vi "GOOP_RecompileDialog.vi"(5 "error in (no error)":errorcluster) -> (19 "error out":errorcluster)   [LabVIEW 2020]
panel:
  out "Progress":u8(slide) scale=0.0..100.0
  in  "_Cancel":bool
  in  "_Recompile":bool
  # "Open GOOP\nDevelopment Suite"
  # "OpenGDS needs to be re-compiled. If you re-compile the OpenGDS it will load faster and be more stable. Do you want to re-compile now?\nIt will take some time to re-compile OpenGDS."
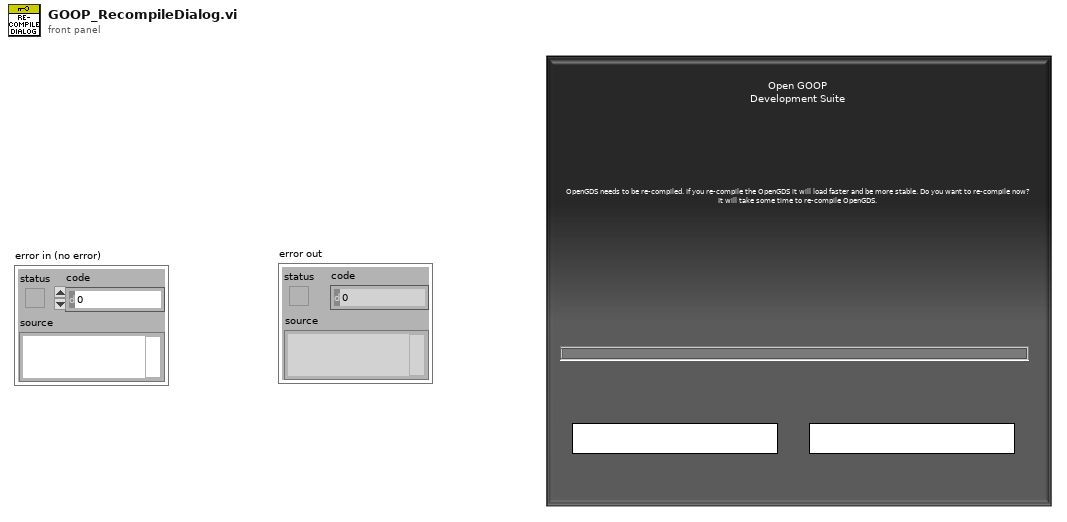
[diagram p1: front panel]
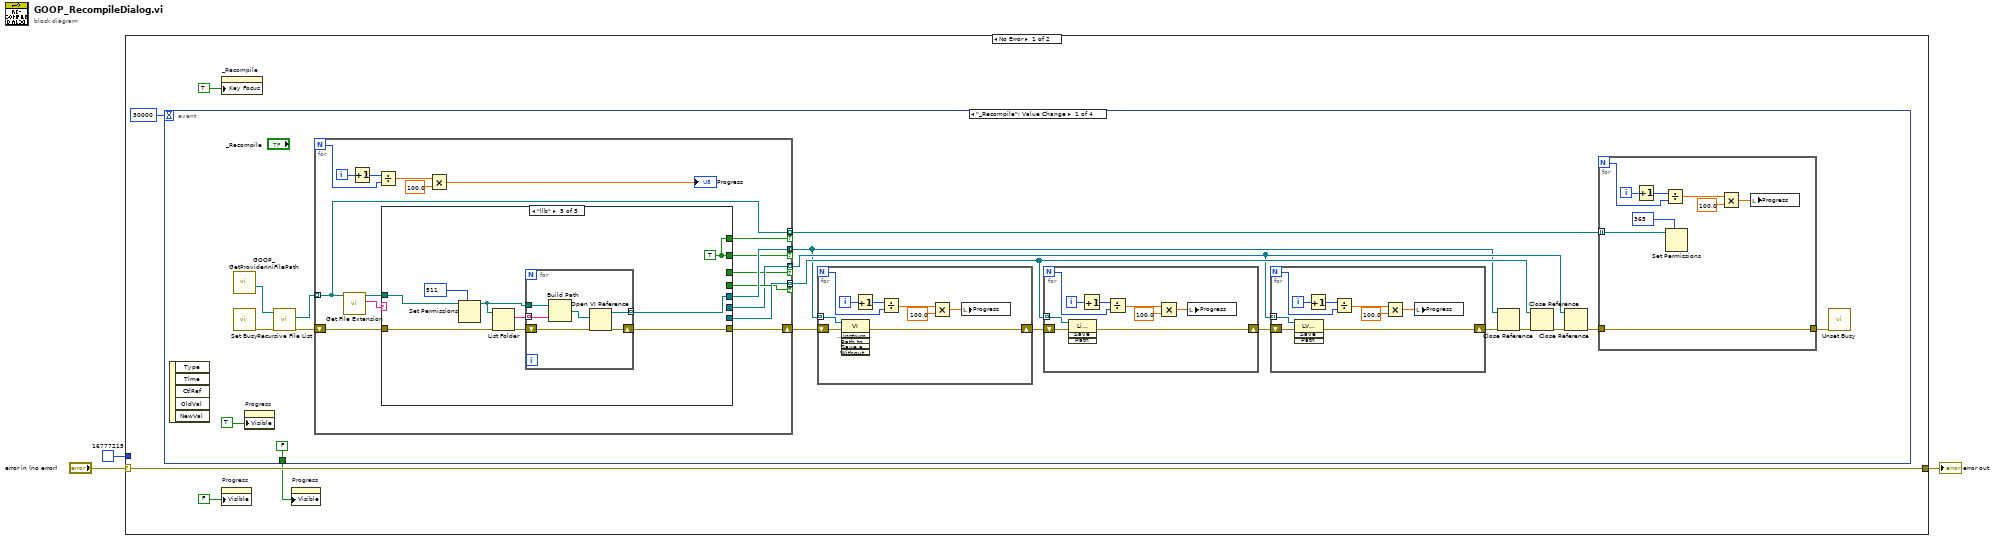
[diagram p0: block diagram]
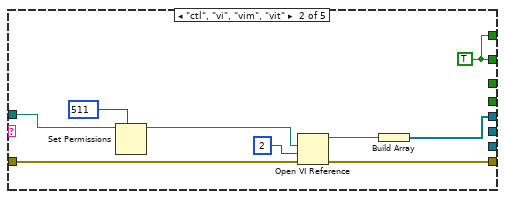
[diagram p3: hidden frame]
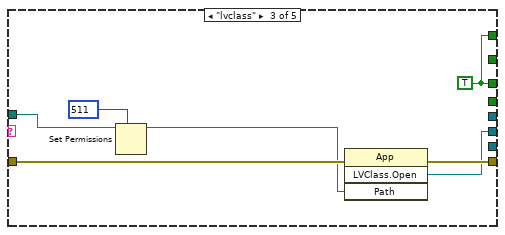
[diagram p4: hidden frame]
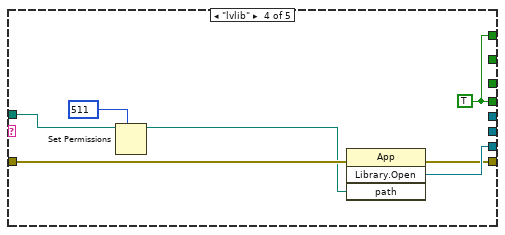
[diagram p5: hidden frame]
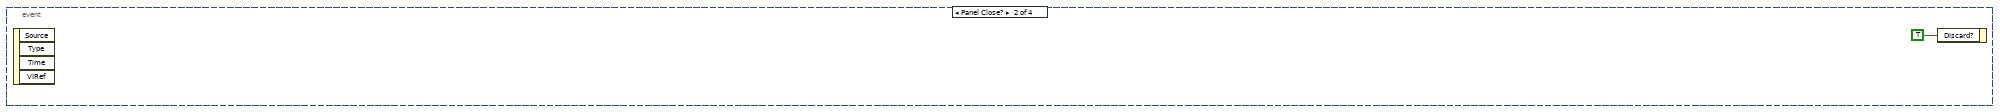
[diagram p6: hidden frame]
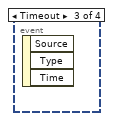
[diagram p7: hidden frame]
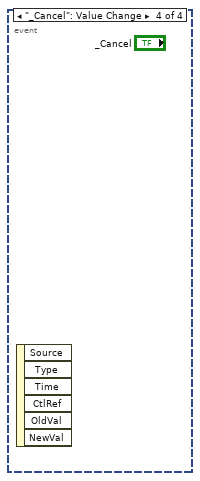
[diagram p8: hidden frame]
diagram:
  n1 = case shown="No Error" "error in (no error)" {
    selector: "error in (no error)" -> [w8 w121]
    tunnel: [w8 w121] -> w3
    tunnel: u32 16777215 -> [_ _]
    frame No Error {
      n2 = event shown="[0] \"_Recompile\": Value Change" {
        selector: _ -> [_ _ _ _]
        dyn-events: _ -> [_ _ _ _]
        timeout: 30000 -> [_ _ _ _]
        tunnel: [FALSE ("Visible") _ _ _] -> w5
        event "_Recompile": Value Change {
          n3 = event-data() -> ()  [unwired: 1 in, 5 out]
          n4 = call <resource>:"GOOP_GetProviderIniFilePath.vi"() -> ("ProviderMainFolder"=w17:path)  [unwired: 10 in, 1 out]
          n5 = call <vilib>:"Set Busy.vi"() -> ("error out"=w12:errorcluster)  [unwired: 10 in, 1 out]
          n6 = property on="Progress" class="Slide (strict)"("Visible"=TRUE) -> ()  [unwired: 2 in, 2 out]
          n7 = call <vilib>:"Recursive File List.vi"("error in (no error)"=w12, "Folder Path"=w17) -> ("error out"=w16:errorcluster, "All Files in Dir"=w15:path[])  [unwired: 5 in, 3 out]
          n8 = for {
            N -> [w67]
            tunnel: [w78] -> w19 mode=concatenating if=w77
            shift-right: [w76] -> w18
            shift-left: w16 -> [w71]
            tunnel: [w75] -> w22 mode=indexing if=w74
            tunnel: [w73] -> w21 mode=indexing if=w72
            tunnel: w15 -> [w70] mode=indexing
            tunnel: [w70] -> w13 mode=indexing if=w69
            i -> [w68]
            n9 = call <vilib>:"Get File Extension.vi"("file"=w70) -> ("lowercase file extension"=w80:string, "dup file"=w79:path)  [unwired: 6 in, 3 out]
            n10 = Increment(x=w68) -> (x+1=w63:i32)
            n11 = Divide(x=w63, y=w67) -> (x/y=w66:dbl)
            n12 = case shown="\"llb\"" w80 {
              tunnel: w71 -> [w81 w90 w97 w104 w109]
              tunnel: w79 -> [_ w84 w93 w100 w107]
              tunnel: [_ w87 _ _ w113] -> w78
              tunnel: [_ w82 _ _ w105] -> w77
              tunnel: [w81 w88 w96 w102 w112] -> w76
              tunnel: [_ _ _ w103 _] -> w75
              tunnel: [_ _ _ w98 _] -> w74
              tunnel: [_ _ w95 _ _] -> w73
              tunnel: [_ _ w91 _ _] -> w72
              tunnel: [_ w82 w91 w98 w105] -> w69
              frame Default {
              }
              frame "ctl", "vi", "vim", "vit" {
                w82 = TRUE
                n13 = Set Permissions(7:i16 511 ("permissions"), 11:w84) -> (3:w83:path)  [unwired: 3 in, 1 out]
                n14 = Open VI Reference(vi path=w83, options=2, error in (no error)=w90) -> (vi reference=w89:refnum<vi>, error out=w88:errorcluster)  [unwired: 3 in]
                n15 = Build Array(w89) -> (w87:refnum<vi>[])
              }
              frame "lvclass" {
                w91 = TRUE
                n16 = Set Permissions(7:i16 511 ("permissions"), 11:w93) -> (3:w92:path)  [unwired: 3 in, 1 out]
                n17 = invoke class="App" method="LVClass.Open"(error in=w97, "Path"=w92) -> (error out=w96:errorcluster, "LVClass.Open"=w95:refnum<vi>)  [unwired: 2 in, 2 out]
              }
              frame "lvlib" {
                w98 = TRUE
                n18 = Set Permissions(7:i16 511 ("permissions"), 11:w100) -> (3:w99:path)  [unwired: 3 in, 1 out]
                n19 = invoke class="App" method="Library.Open"(error in=w104, "path"=w99) -> (error out=w102:errorcluster, "Open Library"=w103:refnum<vi>)  [unwired: 2 in, 2 out]
              }
              frame "llb" {
                w105 = TRUE
                n20 = Set Permissions(7:i16 511 ("permissions"), 11:w107) -> (3:w106:path)  [unwired: 3 in, 1 out]
                n21 = List Folder(path=w106, error in=w109) -> (filenames=w110:string[], error out=w111:errorcluster)  [unwired: 1 in, 3 out]
                n22 = for {
                  tunnel: w110 -> [w114] mode=indexing
                  tunnel: w106 -> [w119]
                  shift-right: [w116] -> w112
                  shift-left: w111 -> [w117]
                  tunnel: [w115] -> w113 mode=indexing
                  n23 = Build Path(base path=w119, name or relative path=w114) -> (appended path=w118:path)
                  n24 = Open VI Reference(vi path=w118, error in (no error)=w117) -> (vi reference=w115:refnum<vi>, error out=w116:errorcluster)  [unwired: 4 in]
                }
              }
            }
            n25 = Multiply(x=w66, y=100.0) -> (x*y=→"Progress":dbl)
          }
          n26 = for {
            N -> [w55]
            tunnel: w19 -> [w62] mode=indexing
            shift-right: [w60] -> w26
            shift-left: w18 -> [w61]
            i -> [w56]
            n27 = invoke class="VI" method="Save.Instrument"(reference=w62, error in=w61) -> (error out=w60:errorcluster)  [unwired: 4 in, 5 out]
            n28 = Increment(x=w56) -> (x+1=w59:i32)
            n29 = Divide(x=w59, y=w55) -> (x/y=w57:dbl)
            n30 = Multiply(x=w57, y=100.0) -> (x*y=w54:dbl)
            n31 = local write "Progress"(w54) -> ()
          }
          n32 = for {
            N -> [w45]
            tunnel: w22 -> [w53] mode=indexing
            shift-right: [w51] -> w25
            shift-left: w26 -> [w52]
            i -> [w46]
            n33 = invoke class="Library" method="Save"(reference=w53, error in=w52) -> (error out=w51:errorcluster)  [unwired: 2 in, 3 out]
            n34 = Increment(x=w46) -> (x+1=w47:i32)
            n35 = Divide(x=w47, y=w45) -> (x/y=w49:dbl)
            n36 = Multiply(x=w49, y=100.0) -> (x*y=w50:dbl)
            n37 = local write "Progress"(w50) -> ()
          }
          n38 = for {
            N -> [w36]
            tunnel: w21 -> [w44] mode=indexing
            shift-right: [w42] -> w24
            shift-left: w25 -> [w43]
            i -> [w37]
            n39 = invoke class="LVClassLibrary" method="Save"(reference=w44, error in=w43) -> (error out=w42:errorcluster)  [unwired: 2 in, 3 out]
            n40 = Increment(x=w37) -> (x+1=w38:i32)
            n41 = Divide(x=w38, y=w36) -> (x/y=w40:dbl)
            n42 = Multiply(x=w40, y=100.0) -> (x*y=w41:dbl)
            n43 = local write "Progress"(w41) -> ()
          }
          n44 = Close Reference(reference=w19, error in (no error)=w24) -> (error out=w23:errorcluster)
          n45 = Close Reference(reference=w22, error in (no error)=w23) -> (error out=w20:errorcluster)
          n46 = Close Reference(reference=w21, error in (no error)=w20) -> (error out=w14:errorcluster)
          n47 = for {
            N -> [w27]
            tunnel: w14 -> [w33]
            tunnel: w13 -> [w34] mode=indexing
            tunnel: [w33] -> w11
            i -> [w28]
            n48 = Increment(x=w28) -> (x+1=w32:i32)
            n49 = Divide(x=w32, y=w27) -> (x/y=w30:dbl)
            n50 = Set Permissions(7:i16 365 ("permissions"), 11:w34) -> ()  [unwired: 3 in, 2 out]
            n51 = Multiply(x=w30, y=100.0) -> (x*y=w29:dbl)
            n52 = local write "Progress"(w29) -> ()
          }
          n53 = call <vilib>:"Unset Busy.vi"("error in (no error)"=w11) -> ()  [unwired: 10 in, 1 out]
        }
        event Panel Close? {
          n54 = event-data() -> ()  [unwired: 1 in, 4 out]
          n55 = event-data("Discard?"=TRUE) -> ()  [unwired: 1 in, 1 out]
        }
        event Timeout {
          n56 = event-data() -> ()  [unwired: 1 in, 3 out]
        }
        event "_Cancel": Value Change {
          n57 = event-data() -> ()  [unwired: 1 in, 6 out]
        }
      }
      n58 = property on="_Recompile" class="Bool"("Key Focus"=TRUE) -> ()  [unwired: 2 in, 2 out]
      n59 = property on="Progress" class="Slide (strict)"("Visible"=FALSE) -> ()  [unwired: 2 in, 2 out]
      n60 = property on="Progress" class="Slide (strict)"("Visible"=w5) -> ()  [unwired: 2 in, 2 out]
    }
    frame Error {
    }
  }
  "error out" <- w3
